vi "PH_AWG-510.PC Get Trigger Settings.vi"(0 "VI in":refnum<vi>, 5 "error in (no error)":errorcluster) -> (14 "VI out":refnum<vi>, 19 "error out":errorcluster)   [LabVIEW 2014, in "PH_AWG-510.lvlib"]
doc: "This VI requests the current trigger settings to store them at own attributes and to tisplay them at the GUI."
uses:
  PH_AWG-510.lvlib
  instr.lib/awg510/Tektronix AWG510.lvlib
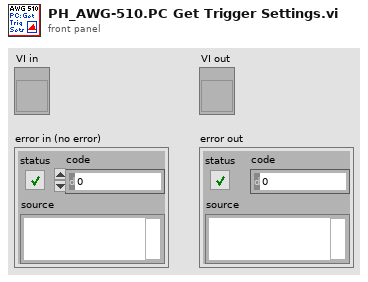
[diagram p1: front panel]
types:
  T1 = typedef "PH_AWG-510.lvlib/PH_AWG-510.i attribute.ctl" = cluster{"GUI Refs":cluster{"Delete":refnum<vi>, "Trigger Settings":refnum<vi>, "Start Device":refnum<vi>, "Instrument Information":refnum<vi>, "Lock Frontpanel":refnum<vi>, "Waveform Pattern File":refnum<vi>, "Initialize":refnum<vi>, "Output Settings":refnum<vi>}, "Instrument Information":T2, "Initialized?":bool, "Current Settings":cluster{"Trigger":T3, "Output Settings":T4}, "Wanted Settings":cluster{"Trigger":T3, "Output Settings":T4}, "Device frontpanel locked?":bool, "Default File Path":path}
  T2 = typedef "PH_AWG-510.lvlib/PH_AWG-510.Instrument Information Dataset.ctl" = cluster{"VISA resource name":refnum<visa-resource-name>, "Instrument Firmware Revision":string, "Manufacturer":string, "Model":string, "Serial Number":string, "Error Message":string, "Device Status":enum16{"stopped", "wating for trigger", "running", "Failure"}}
  T3 = typedef "PH_AWG-510.lvlib/PH_AWG-510.Trigger Settings.ctl" = cluster{"Mode":enum16{"Continuous", "Triggered", "Gated", "Enhanced"}, "Level (V)":dbl, "External Source":bool}
  T4 = typedef "PH_AWG-510.lvlib/PH_AWG-510.Output Settings.ctl" = cluster{"Activate Channel":bool, "VPP (V)":dbl, "Clock (Hz)":dbl, "File Name (Device)":string, "#1":u16, "#2":u16, "#3":u16, "#4":u16, "#5":u16, "#6":u16, "#7":u16, "#8":u16, "#9":u16, "#10":u16, "#11":u16, "#12":u16, "#13":u16, "#14":u16, "#15":u16, "#16":u16, "#17":u16, "#18":u16, "#19":u16, "#20":u16, "Offset (V)":dbl}
  T5 = enum16{"Continuous", "Triggered", "Gated", "Enhanced", "Unknown"}
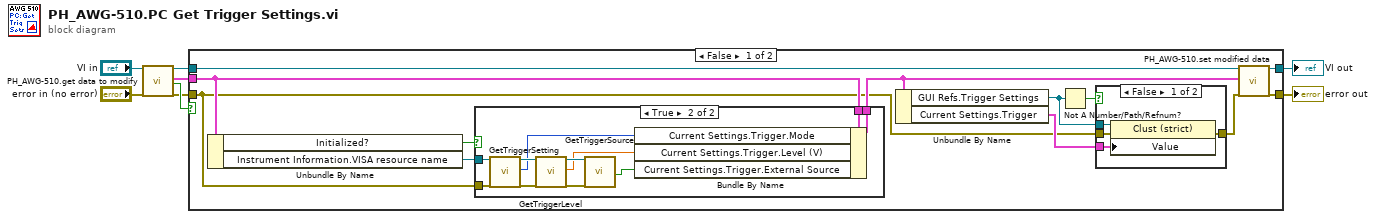
[diagram p0: block diagram]
diagram:
  n1 = call "PH_AWG-510.get data to modify.vi"("i ref in"="VI in", "error in (no error)"="error in (no error)") -> ("i ref out"=w6:refnum<vi>, "i attribute"=w7:T1, "timed out"=w8:bool, "error out"=w4:errorcluster)  [unwired: 14 in]
  n2 = case shown="False" w8 {
    tunnel: w4 -> [w10 w39]
    tunnel: [w20 w39] -> w2
    tunnel: w6 -> [w19 w38]
    tunnel: w7 -> [w17 _]
    tunnel: [w18 w38] -> w1
    frame False {
      n3 = Unbundle By Name(w17) -> ("Initialized?"=w15:bool, "Instrument Information.VISA resource name"=w16:refnum<visa-resource-name>)
      n4 = case shown="True" w15 {
        tunnel: [w26 w37] -> w13
        tunnel: w17 -> [w26 w36]
        tunnel: w16 -> [_ w35]
        tunnel: w10 -> [_ w34]
        frame False {
        }
        frame True {
          n5 = call "GetTriggerSetting.vi"("VISA resource name"=w35, "error in"=w34) -> ("VISA resource name out"=w32:refnum<visa-resource-name>, "Trigger Status"=w29:T5, "error out"=w33:errorcluster)  [unwired: 15 in]
          n6 = call "GetTriggerLevel.vi"("VISA resource name"=w32, "error in"=w33) -> ("VISA resource name out"=w30:refnum<visa-resource-name>, "Trigger Level (V)"=w28:dbl, "error out"=w31:errorcluster)  [unwired: 15 in]
          n7 = call "GetTriggerSource.vi"("VISA resource name"=w30, "error in"=w31) -> ("Trigger source external?"=w27:bool)  [unwired: 15 in, 2 out]
          n8 = Bundle By Name(cluster=w36, "Current Settings.Trigger.Mode"=w29, "Current Settings.Trigger.Level (V)"=w28, "Current Settings.Trigger.External Source"=w27) -> (w37:T1)
        }
      }
      n9 = Unbundle By Name(w13) -> ("GUI Refs.Trigger Settings"=w12:refnum<vi>, "Current Settings.Trigger"=w11:T3)
      n10 = Not A Number/Path/Refnum?(number/path/refnum=w12) -> (NaN/Path/Refnum?=w14:bool)
      n11 = case shown="False" w14 {
        tunnel: w10 -> [w24 w25]
        tunnel: [w23 w25] -> w9
        tunnel: w12 -> [w22 _]
        tunnel: w11 -> [w21 _]
        frame False {
          n12 = property class="Clust (strict)"(reference=w22, error in=w24, "Value"=w21) -> (error out=w23:errorcluster)  [unwired: 1 out]
        }
        frame True {
        }
      }
      n13 = call "PH_AWG-510.set modified data.vi"("i ref in"=w19, "i attribute"=w13, "error in (no error)"=w9) -> ("i ref out"=w18:refnum<vi>, "error out"=w20:errorcluster)  [unwired: 15 in]
    }
    frame True {
    }
  }
  "VI out" <- w1
  "error out" <- w2
